vi "VICI Valve_1.vi"(5 "RequestedValve#":i32) -> (0 "Error? (bool)":bool, 1 "Error?":i32, 2 "Read Position":i32)   [LabVIEW 2019]
panel:
  out "Attempt Iteration":i32
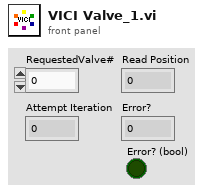
[diagram p1: front panel]
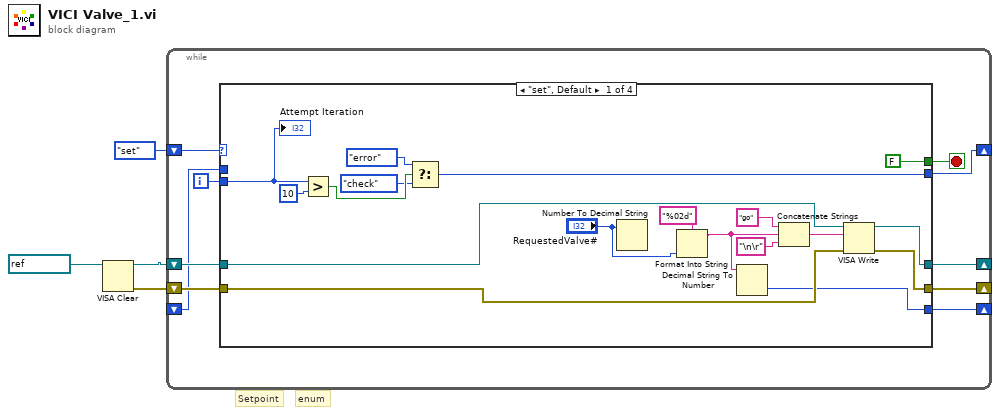
[diagram p0: block diagram]
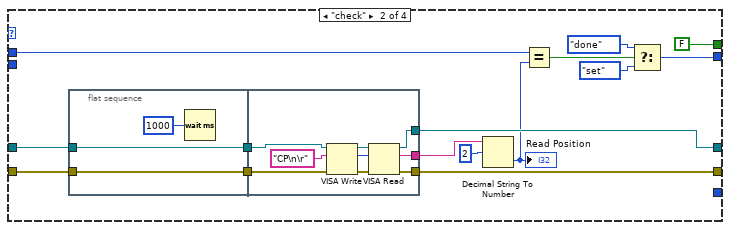
[diagram p2: hidden frame]
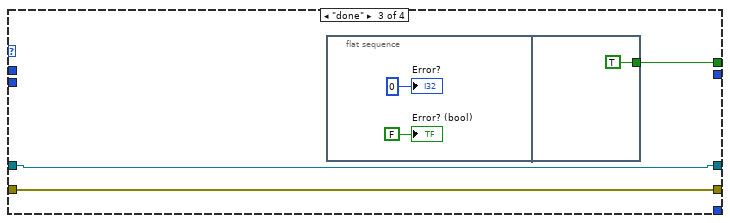
[diagram p3: hidden frame]
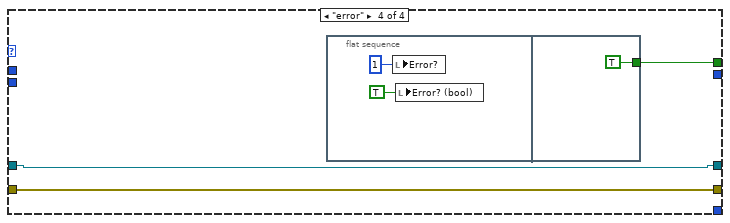
[diagram p4: hidden frame]
diagram:
  # "enum"
  # "Setpoint"
  n1 = VISA Clear(VISA resource name=refnum<visa-resource-name> "COM6") -> (VISA resource name out=w2:refnum<visa-resource-name>, error out=w1:errorcluster)  [unwired: 1 in]
  n2 = while {
    shift-right: [w14] -> _
    shift-left: w1 -> [w12]
    shift-right: [w13] -> _
    shift-left: w2 -> [w11]
    shift-right: [w9] -> _
    shift-left: _ -> [w8]
    shift-right: [w6] -> _
    shift-left: enum16{"set", "check", "done", "error"}."set" -> [w7]
    i -> [w5]
    stop <- w10 stop-if-true
    n3 = case shown="\"set\", Default" w7 {
      tunnel: [w24 w45 w60 w66] -> w14
      tunnel: [w25 w44 w61 w67] -> w13
      tunnel: w12 -> [w32 w42 w60 w66]
      tunnel: w11 -> [w31 w43 w61 w67]
      tunnel: [FALSE FALSE w62 w68] -> w10
      tunnel: [w29 _ _ _] -> w9
      tunnel: w8 -> [_ w41 _ _]
      tunnel: [w23 w36 _ _] -> w6
      tunnel: w5 -> [w22 _ _ _]
      frame "set", Default {
        n4 = Greater?(x=w22, y=10) -> (0:w20:bool)
        n5 = Select(t=enum16{"set", "check", "done", "error"}."error", s=w20, f=enum16{"set", "check", "done", "error"}."check") -> (s? t:f=w23:enum16{"set", "check", "done", "error"})
        n6 = Number To Decimal String(number="RequestedValve#") -> ()  [unwired: 1 in, 1 out]
        n7 = Format Into String(format string="%02d", "RequestedValve#") -> (resulting string=w15:string)  [unwired: 2 in, 1 out]
        n8 = Decimal String To Number(string=w15) -> (number=w29:i32)  [unwired: 2 in, 1 out]
        n9 = Concatenate Strings("go" ("string"), w15, "\n\r" ("string")) -> (w28:string)
        n10 = VISA Write(VISA resource name=w31, write buffer=w28, error in (no error)=w32) -> (VISA resource name out=w25:refnum<visa-resource-name>, error out=w24:errorcluster)  [unwired: 1 out]
        "Attempt Iteration" <- w22
      }
      frame "check" {
        n11 = flat-sequence {
          tunnel: w42 -> [w49]
          tunnel: w43 -> [w50]
          tunnel: [w50] -> w34
          tunnel: [w49] -> w33
          tunnel: [w59] -> w47
          tunnel: [w58] -> w45
          tunnel: [w57] -> w44
          tunnel: w34 -> [w55]
          tunnel: w33 -> [w52]
          frame #0 {
            n12 = Wait (ms)(milliseconds to wait=u32 1000) -> ()  [unwired: 1 out]
          }
          frame #1 {
            n13 = VISA Write(VISA resource name=w55, write buffer="CP\n\r", error in (no error)=w52) -> (VISA resource name out=w54:refnum<visa-resource-name>, return count=w51:u32, error out=w53:errorcluster)
            n14 = VISA Read(VISA resource name=w54, byte count=w51, error in (no error)=w53) -> (VISA resource name out=w57:refnum<visa-resource-name>, read buffer=w59:string, error out=w58:errorcluster)  [unwired: 1 out]
          }
        }
        n15 = Decimal String To Number(string=w47, offset=2) -> (number=w40:i32)  [unwired: 1 in, 1 out]
        "Read Position" <- w40
        n16 = Equal?(x=w41, y=w40) -> (x = y?=w39:bool)
        n17 = Select(t=enum16{"set", "check", "done", "error"}."done", s=w39, f=enum16{"set", "check", "done", "error"}."set") -> (s? t:f=w36:enum16{"set", "check", "done", "error"})
      }
      frame "done" {
        n18 = flat-sequence {
          tunnel: [TRUE] -> w62
          frame #0 {
            "Error?" <- 0
            "Error? (bool)" <- FALSE
          }
          frame #1 {
          }
        }
      }
      frame "error" {
        n19 = flat-sequence {
          tunnel: [TRUE] -> w68
          frame #0 {
            n20 = local write "Error?"(1) -> ()
            n21 = local write "Error? (bool)"(TRUE) -> ()
          }
          frame #1 {
          }
        }
      }
    }
  }
